vi "Configure FFT Measurement Result Rejection.vi"(8 "error in (no error)":errorcluster, 9 "Measure on Exception (Off)":bool, 10 "Instance (1)":i32=1, 11 "VISA resource name":refnum<visa-resource-name>) -> (0 "error out":errorcluster, 3 "VISA resource name out":refnum<visa-resource-name>)   [LabVIEW 2020, in "Rohde&Schwarz CMXP GPRF.lvlib"]
doc: "Specifies whether measurement results that the R&S CMW identifies as faulty or inaccurate are rejected.\n\nAttribute:\nRSCMXPGPRF_ATTR_FFT_MEASUREMENT_RESULTS_REJECTION\n\nRemote-control command:\nCONFigure:GPRF:MEAS<i>:FFTSanalyzer:MOEXception"
uses:
  <instrlib>/Rohde&Schwarz CMXP GPRF/Rohde&Schwarz CMXP GPRF.lvlib
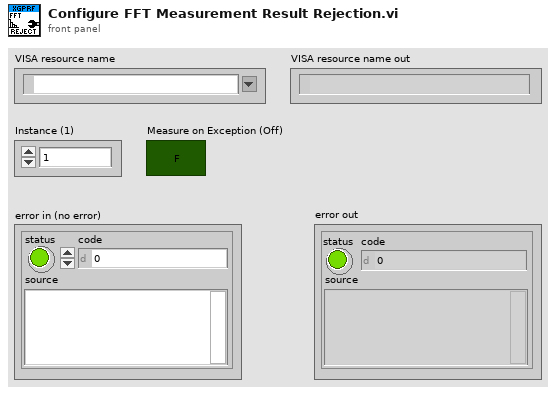
[diagram p1: front panel]
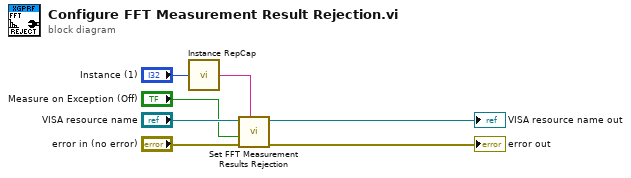
[diagram p0: block diagram]
diagram:
  n1 = call <instrlib>:"Instance RepCap.vi"("Instance in"="Instance (1)") -> ("Instance out"=w7:string)
  n2 = call "Set FFT Measurement Results Rejection"("Repeated Capabilities"=w7, "error in (no error)"="error in (no error)", "FFT Measurement Results Rejection (OFF)"="Measure on Exception (Off)", "instrument handle"="VISA resource name") -> ("error out"=→"error out":errorcluster, "instrument handle out"=→"VISA resource name out":refnum<visa-resource-name>)  [unwired: 6 in]
